vi "test variant to json enum.vi"(8 "error in (no error)":errorcluster) -> (0 "error out":errorcluster)   [LabVIEW 2019, in "labview_json_tests.lvlib"]
uses:
  labview_json_tests.lvlib
  lib/labview_json.lvlib
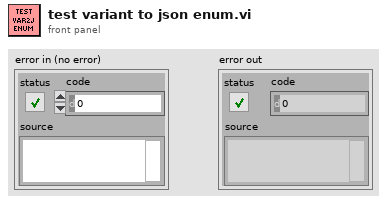
[diagram p1: front panel]
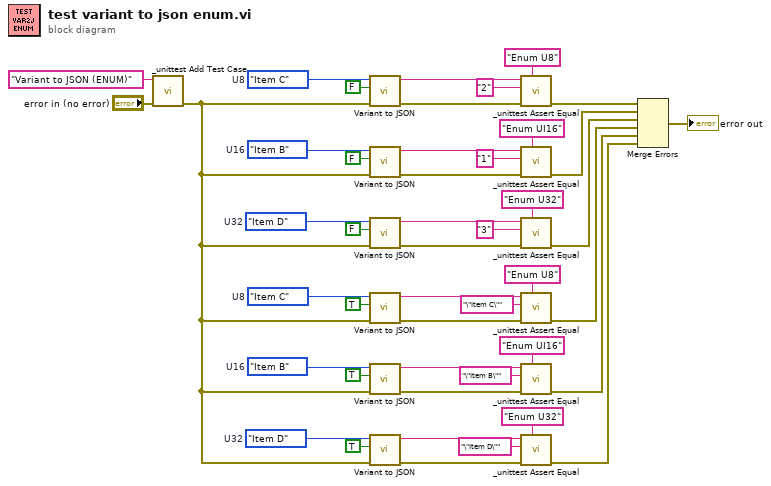
[diagram p0: block diagram]
diagram:
  w21 = enum32{"Item A", "Item B", "Item C", "Item D"}."Item D"  # U32
  w4 = enum16{"Item A", "Item B", "Item C", "Item D"}."Item B"  # U16
  w18 = enum8{"Item A", "Item B", "Item C", "Item D"}."Item C"  # U8
  w24 = enum32{"Item A", "Item B", "Item C", "Item D"}."Item D"  # U32
  w26 = enum16{"Item A", "Item B", "Item C", "Item D"}."Item B"  # U16
  w28 = enum8{"Item A", "Item B", "Item C", "Item D"}."Item C"  # U8
  n1 = call "_unittest Add Test Case.vi"("error in (no error)"="error in (no error)", "Test Case"="Variant to JSON (ENUM)") -> ("error out"=w5:errorcluster)  [unwired: 9 in]
  n2 = call "Variant to JSON.vi"("error in (no error)"=w5, "Enums as string? (F)"=FALSE, "Variant in"=w28) -> ("error out"=w39:errorcluster, "JSON"=w38:string)  [unwired: 7 in]
  n3 = call "Variant to JSON.vi"("error in (no error)"=w5, "Enums as string? (F)"=FALSE, "Variant in"=w26) -> ("error out"=w37:errorcluster, "JSON"=w36:string)  [unwired: 7 in]
  n4 = call "Variant to JSON.vi"("error in (no error)"=w5, "Enums as string? (F)"=FALSE, "Variant in"=w24) -> ("error out"=w31:errorcluster, "JSON"=w32:string)  [unwired: 7 in]
  n5 = call "Variant to JSON.vi"("error in (no error)"=w5, "Enums as string? (F)"=TRUE, "Variant in"=w18) -> ("error out"=w8:errorcluster, "JSON"=w9:string)  [unwired: 7 in]
  n6 = call "Variant to JSON.vi"("error in (no error)"=w5, "Enums as string? (F)"=TRUE, "Variant in"=w4) -> ("error out"=w10:errorcluster, "JSON"=w11:string)  [unwired: 7 in]
  n7 = call "Variant to JSON.vi"("error in (no error)"=w5, "Enums as string? (F)"=TRUE, "Variant in"=w21) -> ("error out"=w16:errorcluster, "JSON"=w15:string)  [unwired: 7 in]
  n8 = call "_unittest Assert Equal.vi"("Message"="Enum U8", "error in (no error)"=w39, "Expected Value"="2", "Actual Value"=w38) -> ("error out"=w44:errorcluster)  [unwired: 7 in]
  n9 = call "_unittest Assert Equal.vi"("Message"="Enum UI16", "error in (no error)"=w37, "Expected Value"="1", "Actual Value"=w36) -> ("error out"=w40:errorcluster)  [unwired: 7 in]
  n10 = call "_unittest Assert Equal.vi"("Message"="Enum U32", "error in (no error)"=w31, "Expected Value"="3", "Actual Value"=w32) -> ("error out"=w29:errorcluster)  [unwired: 7 in]
  n11 = call "_unittest Assert Equal.vi"("Message"="Enum U8", "error in (no error)"=w8, "Expected Value"="\"Item C\"", "Actual Value"=w9) -> ("error out"=w3:errorcluster)  [unwired: 7 in]
  n12 = call "_unittest Assert Equal.vi"("Message"="Enum UI16", "error in (no error)"=w10, "Expected Value"="\"Item B\"", "Actual Value"=w11) -> ("error out"=w2:errorcluster)  [unwired: 7 in]
  n13 = call "_unittest Assert Equal.vi"("Message"="Enum U32", "error in (no error)"=w16, "Expected Value"="\"Item D\"", "Actual Value"=w15) -> ("error out"=w1:errorcluster)  [unwired: 7 in]
  n14 = Merge Errors(w44, w40, w29, w3, w2, w1) -> (→"error out":errorcluster)
